vi "Remove SubPanel.vi"(11 "Subpanel Ref":refnum<vi>) -> (0 "error out":errorcluster)   [LabVIEW 2021, in "Model.lvlib"]
uses:
  Model.lvlib
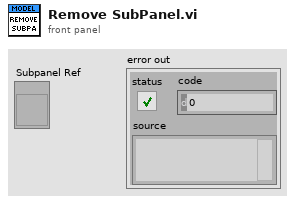
[diagram p1: front panel]
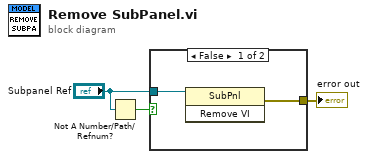
[diagram p0: block diagram]
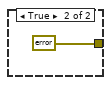
[diagram p2: hidden frame]
diagram:
  n1 = Not A Number/Path/Refnum?(number/path/refnum="Subpanel Ref") -> (NaN/Path/Refnum?=w3:bool)
  n2 = case shown="False" w3 {
    tunnel: "Subpanel Ref" -> [w4 _]
    tunnel: [w5 errorcluster {"status"=FALSE, "code"=0, "source"=""} ("error out")] -> w1
    frame False {
      n3 = invoke on="Invoke Node" class="SubPnl" method="Remove VI"(reference=w4) -> (error out=w5:errorcluster)  [unwired: 2 in, 2 out]
    }
    frame True {
    }
  }
  "error out" <- w1
